vi "Set Stream and Connection.vi"(8 "error in (no error)":errorcluster, 9 "Stream":refnum<class "WebsocketStream.lvclass">, 10 "TCP Connection":refnum<k5>, 11 "Websocket Client in":refnum<class "Websocket Client.lvclass">) -> (0 "error out":errorcluster, 3 "Websocket Client out":refnum<class "Websocket Client.lvclass">)   [LabVIEW 2020, in "Stream-Websocket.lvlib" / "Websocket Client.lvclass"]
uses:
  Websocket Client.lvclass
  WebsocketStream/WebsocketStream.lvclass
  Websocket Client.lvclass/Websocket Client.ctl
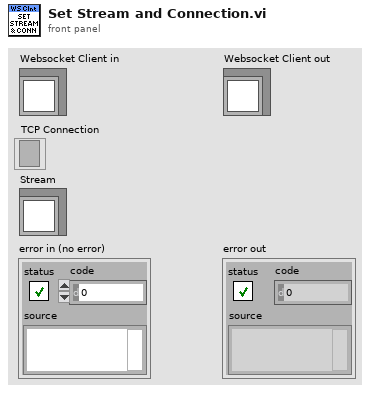
[diagram p1: front panel]
types:
  T1 = typedef "Stream-Websocket.lvlib/Websocket Client.lvclass/Ref Data.ctl" = cluster{"TCP Connection":refnum<k5>, "WS Stream":refnum<class "WebsocketStream.lvclass">, "Connection Loop":refnum<vi>, "Timeout ms":i32, "Server Connection":bool}
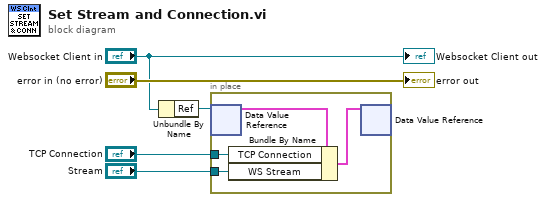
[diagram p0: block diagram]
diagram:
  n1 = Unbundle By Name("Websocket Client in") -> ("Ref"=w4:refnum<data-value>)
  n2 = in-place {
    in-place-border: "TCP Connection" -> [w7]
    in-place-border: "Stream" -> [w6]
    n3 = in-place-dvr #1(w4) -> (w9:T1)  [unwired: 1 out]
    n4 = Bundle By Name(cluster=w9, "TCP Connection"=w7, "WS Stream"=w6) -> (w8:T1)
    n5 = in-place-dvr #1(w8) -> ()  [unwired: 2 out]
  }
  "error out" <- "error in (no error)"
  "Websocket Client out" <- "Websocket Client in"
